vi "PID Test Y-axis.vi"() -> ()   [LabVIEW 2017]
uses:
  <vilib>/myRIO/Common/Instrument Driver Framework/myRIO v1.0/UART/vis/myRIO v1.0 Close UART.vi
  <vilib>/addons/control/pid/pid.llb/PID Control Input Filter (DBL).vi
  <vilib>/addons/control/pid/pid.llb/PID (DBL).vi
  <vilib>/myRIO/Common/Instrument Driver Framework/Utilities/vis/FPGA Ref Manager.vi
  <vilib>/myRIO/Common/Instrument Driver Framework/myRIO v1.0/myRIO v1.0 Reset FPGA.vi
  <vilib>/myRIO/Common/Instrument Driver Framework/myRIO v1.0/IRQ/vis/myRIO v1.0 IRQ Info FGV.vi
  <vilib>/myRIO/Common/Instrument Driver Framework/myRIO v1.0/IRQ/vis/myRIO v1.0 Timer IRQ Info FGV.vi
  <vilib>/myRIO/Common/Instrument Driver Framework/myRIO v1.0/IRQ/vis/myRIO v1.0 ISR Agent.vi
  <vilib>/addons/control/pid/NI_PID_pid.lvlib
  <vilib>/myRIO/Instrument Drivers/Utilities/Utilities.lvlib
  <vilib>/ptbypt/NI_PtbyPt.lvlib
panel:
  out "Sensor Output":cluster{dbl, "output":dbl}(graph)
  out "Motion Data":T1
  in  "FWD/RVS":bool
  out "Time (s)":dbl
  out "Output String":string
  out "PID Output":dbl(graph)
  out "SP & PV":T2(graph)
  in  "PID gains":T3={"proportional gain (Kc)"=1.0, "integral time (Ti, min)"=0.01, "derivative time (Td, min)"=0.0} {"derivative time (Td, min)" format="%.6f"; "integral time (Ti, min)" format="%.6f"; "proportional gain (Kc)" format="%.3f"}
  in  "Velocity Set Pt":dbl
  in  "stop":bool
  # "15mm/s  max"
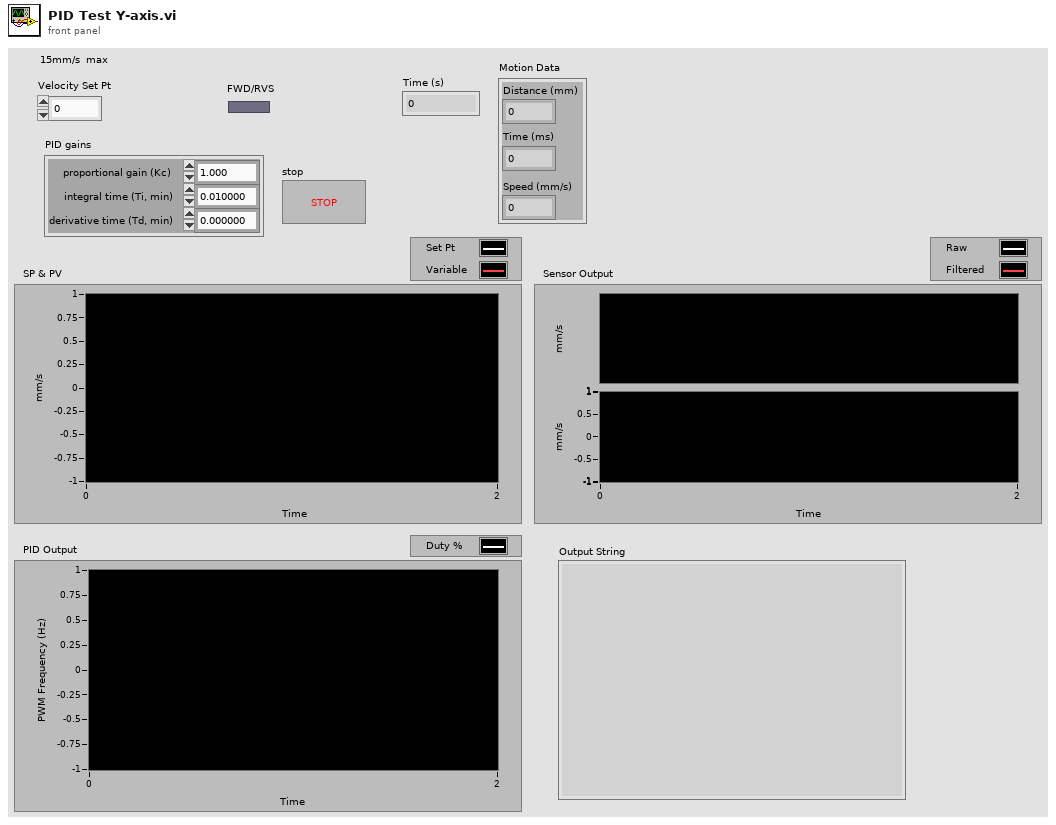
[diagram p1: front panel]
types:
  T1 = cluster{"Distance (mm)":dbl, "Time (ms)":u32, "Speed (mm/s)":dbl}
  T2 = cluster{"Velocity Set Pt":dbl, "Velocity (mm/s)":dbl}
  T3 = cluster{"proportional gain (Kc)":dbl, "integral time (Ti, min)":dbl, "derivative time (Td, min)":dbl}
  T4 = cluster{"Velocity Set Pt":dbl, "Velocity (mm/s)":dbl}[]
  T5 = typedef "Encoder Cluster.ctl" = cluster{"Y-axis rev count":dbl, "Y-axis distance":dbl, "X-axis rev count":dbl, "X-axis distance":dbl, "Y-axis direction":T6, "X-axis direction":T6, "X-counter val":i32, "Y-counter val":i32}
  T6 = typedef "Encoder Count Direction Enum.ctl" = enum16{"Counting Up", "Counting Down"}
  T7 = cluster{dbl, "mean":dbl, dbl, "output":dbl, "proportional gain (Kc)":dbl, "integral time (Ti, min)":dbl, "derivative time (Td, min)":dbl, dbl}
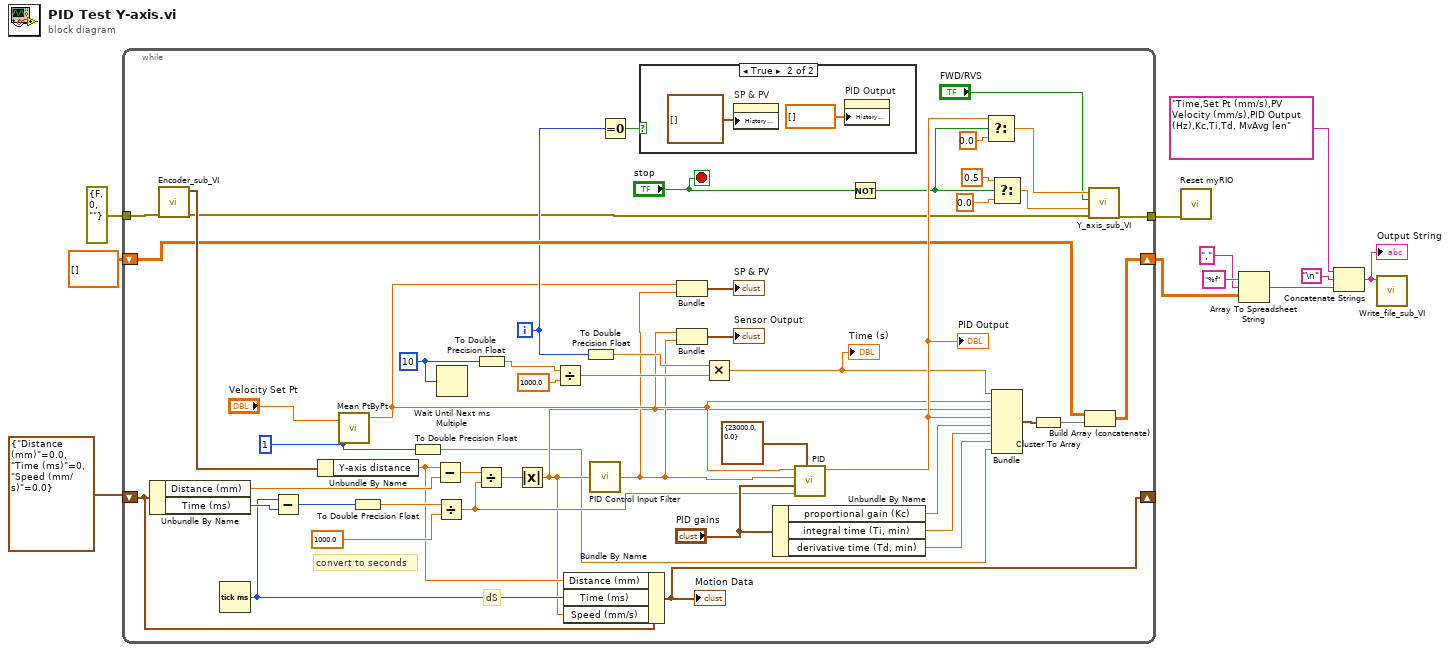
[diagram p0: block diagram]
diagram:
  n1 = while {
    shift-right: [w47] -> w4
    shift-left: dbl[][] [] ("element") -> [w48]
    tunnel: errorcluster {"status"=FALSE, "code"=0, "source"=""} ("error constant") -> [w46]
    tunnel: [w26] -> w2
    shift-right: [w29] -> _
    shift-left: T1 {"Distance (mm)"=0.0, "Time (ms)"=0, "Speed (mm/s)"=0.0} ("Motion Data") -> [w33]
    i -> [w35]
    stop <- "stop" stop-if-true
    w14 = 1 ("sample length")
    w37 = u32 10 ("millisecond multiple")
    # "dS"
    # "convert to seconds"
    n2 = Unbundle By Name(w33) -> ("Distance (mm)"=w34:dbl, "Time (ms)"=w31:u32)
    n3 = call "Encoder_sub_VI.vi"("error in (no error)"=w46) -> ("error out"=w25:errorcluster, "Encoder Output"=w61:T5)  [unwired: 9 in]
    n4 = Tick Count (ms)() -> (millisecond timer value=w30:u32)
    n5 = Subtract(x=w30, y=w31) -> (x-y=w53:u32)
    n6 = Unbundle By Name(w61) -> ("Y-axis distance"=w32:dbl)
    n7 = call <vilib>:"Mean PtByPt.vi"("x"="Velocity Set Pt", "sample length"=w14) -> ("mean"=w17:dbl)  [unwired: 2 in, 1 out]
    n8 = To Double Precision Float(number=w53) -> (double precision float=w52:dbl)
    n9 = To Double Precision Float(number=w14) -> (double precision float=w12:dbl)
    n10 = Subtract(x=w32, y=w34) -> (x-y=w59:dbl)
    n11 = Divide(x=w52, y=1000.0) -> (x/y=w28:dbl)
    n12 = Wait Until Next ms Multiple(millisecond multiple=w37) -> ()  [unwired: 1 out]
    n13 = Divide(x=w59, y=w28) -> (x/y=w58:dbl)
    n14 = To Double Precision Float(number=w37) -> (double precision float=w45:dbl)
    n15 = Absolute Value(x=w58) -> (abs(x)=w15:dbl)
    n16 = Divide(x=w45, y=1000.0) -> (x/y=w40:dbl)
    n17 = Bundle By Name(cluster=w33, "Distance (mm)"=w32, "Time (ms)"=w30, "Speed (mm/s)"=w15) -> (w29:T1)
    "Motion Data" <- w29
    n18 = To Double Precision Float(number=w35) -> (double precision float=w38:dbl)
    n19 = call-poly <vilib>:"PID Control Input Filter.vi"("input"=w15) -> ("output"=w16:dbl)  [unwired: 4 in]
    n20 = Equal To 0?(x=w35) -> (x = 0?=w36:bool)
    n21 = case shown="True" w36 {
      frame False {
      }
      frame True {
        n22 = property on="SP & PV" class="WFChart (strict)"("History Data"=T4 []) -> ()  [unwired: 2 in, 2 out]
        n23 = property on="PID Output" class="WFChart (strict)"("History Data"=dbl[] []) -> ()  [unwired: 2 in, 2 out]
      }
    }
    n24 = Bundle("mean"=w17, "output"=w16) -> (→"SP & PV":cluster{"mean":dbl, "output":dbl})  [unwired: 1 in]
    n25 = Bundle(w15, "output"=w16) -> (→"Sensor Output":cluster{dbl, "output":dbl})  [unwired: 1 in]
    n26 = Multiply(x=w38, y=w40) -> (x*y=w39:dbl)
    "Time (s)" <- w39
    n27 = Unbundle By Name("PID gains") -> ("proportional gain (Kc)"=w43:dbl, "integral time (Ti, min)"=w42:dbl, "derivative time (Td, min)"=w41:dbl)
    n28 = call-poly <vilib>:"PID.vi"("output range"=cluster{"output high":dbl, "output low":dbl} {"output high"=23000.0, "output low"=0.0}, "dt (s)"=w28, "PID gains"="PID gains", "process variable"=w16, "setpoint"=w17) -> ("output"=w51:dbl)  [unwired: 5 in, 1 out]
    "PID Output" <- w51
    n29 = Not(x="stop") -> (.not. x?=w22:bool)
    n30 = Select(t=w51, s=w22, f=0.0) -> (s? t:f=w24:dbl)
    n31 = Select(t=0.5, s=w22, f=0.0) -> (s? t:f=w21:dbl)
    n32 = Bundle(w39, "mean"=w17, w15, "output"=w51, "proportional gain (Kc)"=w43, "integral time (Ti, min)"=w42, "derivative time (Td, min)"=w41, w12) -> (w13:T7)  [unwired: 1 in]
    n33 = Cluster To Array(cluster=w13) -> (array=w49:dbl[])
    n34 = Build Array (concatenate)(w48, w49) -> (w47:dbl[][])
    n35 = call "Y_axis_sub_VI.vi"("error in (no error)"=w25, "Duty Cycle"=w21, "FWD/RVS"="FWD/RVS", "Frequency"=w24) -> ("error out"=w26:errorcluster)  [unwired: 7 in]
  }
  n36 = call <vilib>:"Reset myRIO.vi"("error in (no error)"=w2) -> ()  [unwired: 10 in, 1 out]
  n37 = Array To Spreadsheet String(delimiter (Tab)=",", array=w4, 3:"%f" ("format string")) -> (spreadsheet string=w10:string)
  n38 = Concatenate Strings("Time,Set Pt (mm/s),PV Velocity (mm/s),PID Output (Hz),Kc,Ti,Td, MvAvg len", "\n", w10) -> (w9:string)
  "Output String" <- w9
  n39 = call "Write_file_sub_VI.vi"("Output String"=w9) -> ()  [unwired: 9 in, 2 out]
